vi "氨氮通讯.vi"() -> ()   [LabVIEW 2016, in "氨氮.lvlib"]
uses:
  <vilib>/Utility/config.llb/Write Key (Boolean).vi
  <vilib>/Utility/config.llb/Write Key (String).vi
  <vilib>/Utility/config.llb/Read Key (Boolean).vi
  <vilib>/Utility/config.llb/Read Key (String).vi
  <vilib>/Plasmionique/MB Master/MB_Master/MB_Master.lvclass
  <vilib>/Utility/config.llb/NI_LVConfig.lvlib
  <vilib>/Plasmionique/MB Master/MB Master.lvlib
  <vilib>/ptbypt/NI_PtbyPt.lvlib
panel:
  out "序列号":string
  out "状态告警区":T1
  out "测量数据区":T2 {"单位" items=["ug/L", "mg/L", "ppm", "mg/m3", "cm", "ppb", "ug/m3", "%", "nmol/mol", "umol/mol", "MPN/L", "MPN/100ml", "ng/m3", "NTU", "无量纲", "ms/cm", "us/cm", "℃", "mV", "万个/L"]}
  out "status":bool
  out "关键参数区":T3
  in  "读关键参数区":bool
  in  "读状态告警区":bool
  in  "读测量数据区":bool
  in  "站号":u16(ring) items=["总磷"=1, "氨氮"=3]
  in  "停止":bool
  in  "启动":bool
  in  "控制命令":u16(ring) items=["启动测量"=1, "标样核查"=2, "零点核查"=3, "跨度核查"=4, "空白测试"=5, "平行样测试"=6, "加标回收"=7, "空白校准"=8, "标样校准"=9, "初始化（清洗）"=10, "停止测试"=11, "仪器重启"=12, "校时"=13, "模式设置"=14, "测量间隔设置"=15]
  in  "控制命令参数":u16[](array[numeric]) format="%04xH"
  in  "VISA Resource":refnum<visa-resource-name>
  in  "启用模块":bool
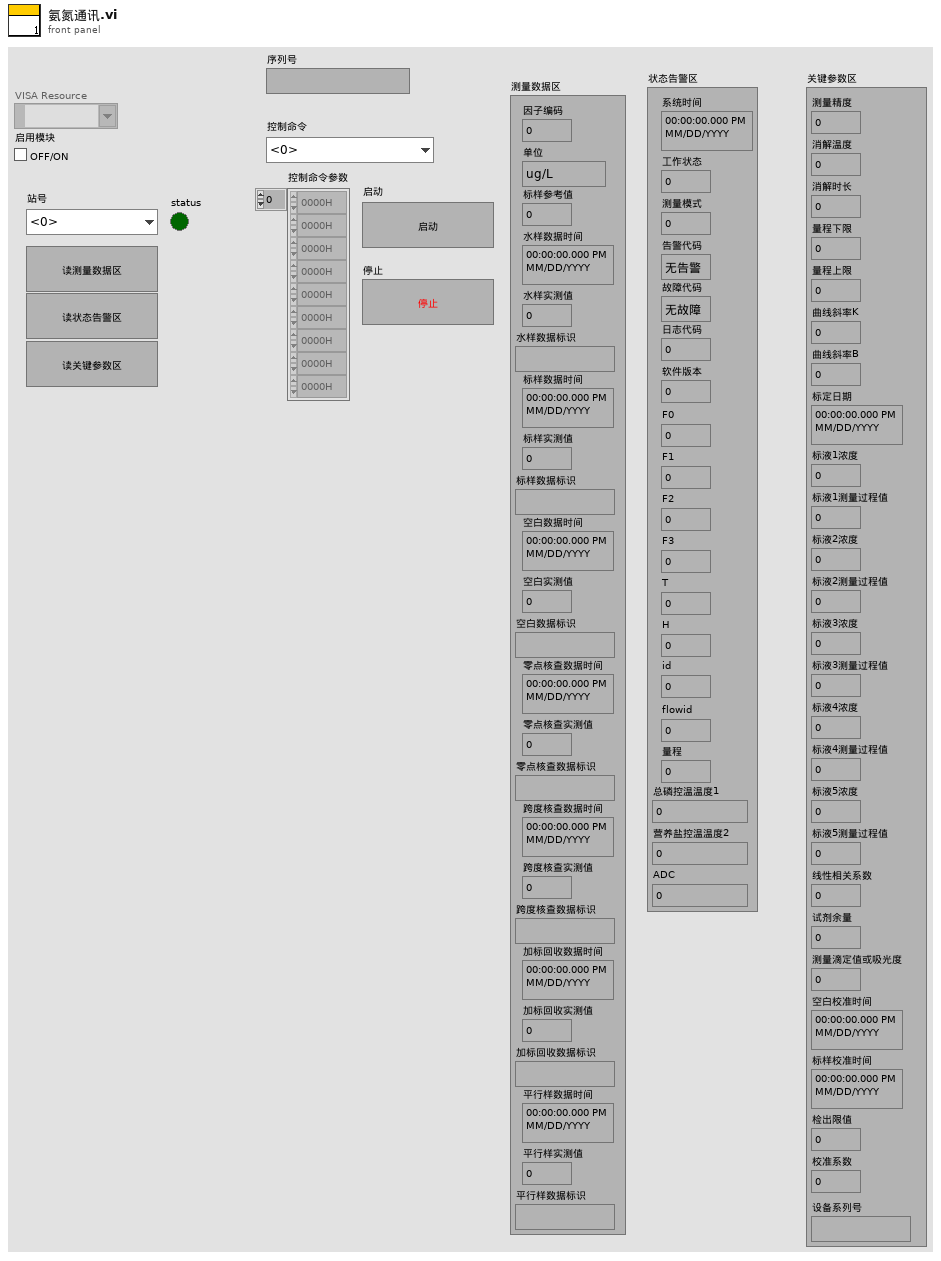
[diagram p1: front panel]
types:
  T1 = cluster{"系统时间":timestamp, "工作状态":u16, "测量模式":u16, "告警代码":enum16{"无告警", "缺试剂告警", "缺水样告警", "缺蒸馏水告警", "缺标液告警", "仪表漏液告警", "标定异常告警", "超量程告警", "加热异常", "低试剂预警", "超上限告警", "超下限告警", "仪表内部其他异常", "滴定异常告警", "电极异常告警", "量程切换告警", "参数设置告警", "PH电极电位异常", "电导率电极异常", "浊度光度异常", "溶解氧电极异常", "溶解氧光强异常", "温度异常告警", "PH异常告警", "溶解氧异常告警", "电导率异常告警", "浊度异常告警", "叶绿素异常告警", "藻密度异常告警", "蓝绿藻异常告警", "ORP异常告警", "氨氮异常告警", "清洁刷异常告警", "SD卡异常告警", "蓝牙异常告警", "Wifi异常告警", "流程异常告警"}, "故障代码":enum16{"无故障", "电机故障", "温度故障", "通讯故障", "滴定故障"}, "日志代码":u16, "软件版本":u16, "F0":sgl, "F1":sgl, "F2":sgl, "F3":sgl, "T":sgl, "H":sgl, "id":u16, "flowid":u16, "量程":u16, "ADC":sgl, "营养盐控温温度2":sgl, "总磷控温温度1":sgl}
  T2 = cluster{"因子编码":u32, "单位":u16, "标样参考值":sgl, "水样数据时间":timestamp, "水样实测值":sgl, "水样数据标识":string, "标样数据时间":timestamp, "标样实测值":sgl, "标样数据标识":string, "空白数据时间":timestamp, "空白实测值":sgl, "空白数据标识":string, "零点核查数据时间":timestamp, "零点核查实测值":sgl, "零点核查数据标识":string, "跨度核查数据时间":timestamp, "跨度核查实测值":sgl, "跨度核查数据标识":string, "加标回收数据时间":timestamp, "加标回收实测值":sgl, "加标回收数据标识":string, "平行样数据时间":timestamp, "平行样实测值":sgl, "平行样数据标识":string}
  T3 = cluster{"测量精度":u16, "消解温度":u16, "消解时长":u16, "量程下限":sgl, "量程上限":sgl, "曲线斜率K":sgl, "曲线斜率B":sgl, "标定日期":timestamp, "标液1浓度":sgl, "标液1测量过程值":sgl, "标液2浓度":sgl, "标液2测量过程值":sgl, "标液3浓度":sgl, "标液3测量过程值":sgl, "标液4浓度":sgl, "标液4测量过程值":sgl, "标液5浓度":sgl, "标液5测量过程值":sgl, "线性相关系数":sgl, "试剂余量":u32, "测量滴定值或吸光度":sgl, "空白校准时间":timestamp, "标样校准时间":timestamp, "检出限值":sgl, "校准系数":sgl, "设备系列号":string}
  T4 = typedef "NI_LVConfig.lvlib/Config Data RefNum.ctl" = refnum<k1>
  T5 = enum8{"Enabled", "Disabled", "Disabled and Grayed Out"}
  T6 = cluster{"系统时间":timestamp, "工作状态":enum16{"空闲", "水样测试", "标样核查", "零点核查", "跨度核查", "空白测试", "平行样测试", "加标回收", "空白校准", "标样校准", "初始化（清洗）"}, "测量模式":enum16{"待机", "连续模式", "周期模式", "定点模式", "受控模式", "手动模式"}, "告警代码":enum16{"无告警", "缺试剂告警", "缺水样告警", "缺蒸馏水告警", "缺标液告警", "仪表漏液告警", "标定异常告警", "超量程告警", "加热异常", "低试剂预警", "超上限告警", "超下限告警", "仪表内部其他异常", "滴定异常告警", "电极异常告警", "量程切换告警", "参数设置告警", "PH电极电位异常", "电导率电极异常", "浊度光度异常", "溶解氧电极异常", "溶解氧光强异常", "温度异常告警", "PH异常告警", "溶解氧异常告警", "电导率异常告警", "浊度异常告警", "叶绿素异常告警", "藻密度异常告警", "蓝绿藻异常告警", "ORP异常告警", "氨氮异常告警", "清洁刷异常告警", "SD卡异常告警", "蓝牙异常告警", "Wifi异常告警", "流程异常告警"}, "故障代码":enum16{"无故障", "电机故障", "温度故障", "通讯故障", "滴定故障"}, "日志代码":u16, "软件版本":u16, "F0":sgl, "F1":sgl, "F2":sgl, "F3":sgl, "T":sgl, "H":sgl, "id":u16, "flowid":u16, "量程":u16, "总磷控温温度1":sgl, "营养盐控温温度2":sgl, "ADC":sgl}
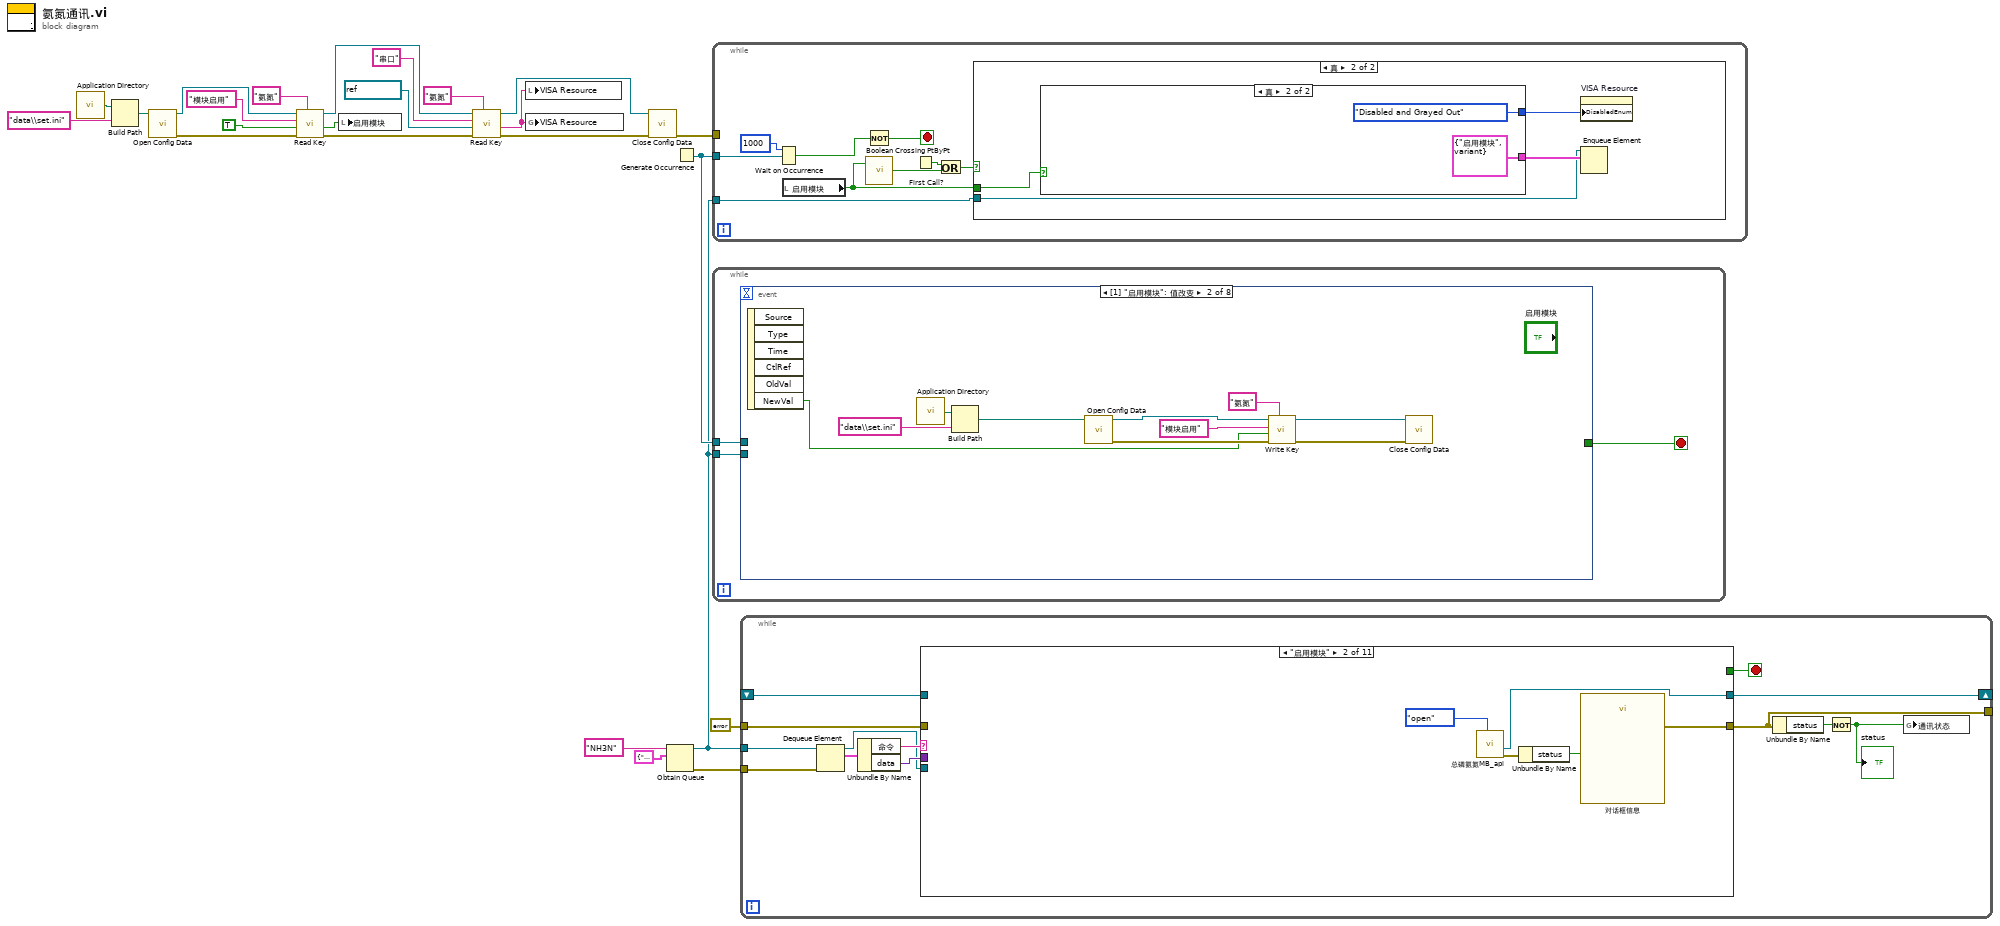
[diagram p0: block diagram]
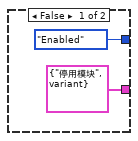
[diagram p3: hidden frame]
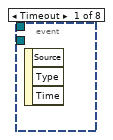
[diagram p4: hidden frame]
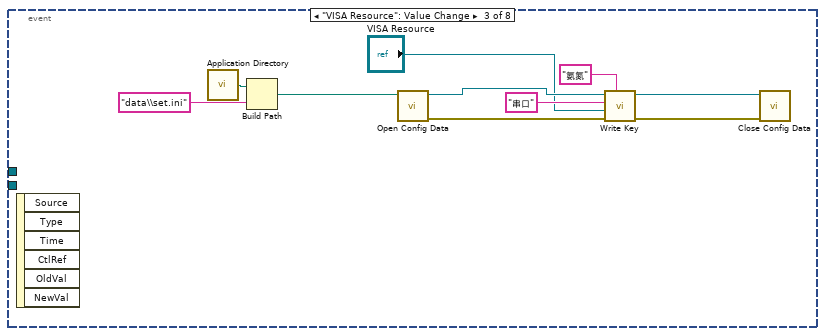
[diagram p5: hidden frame]
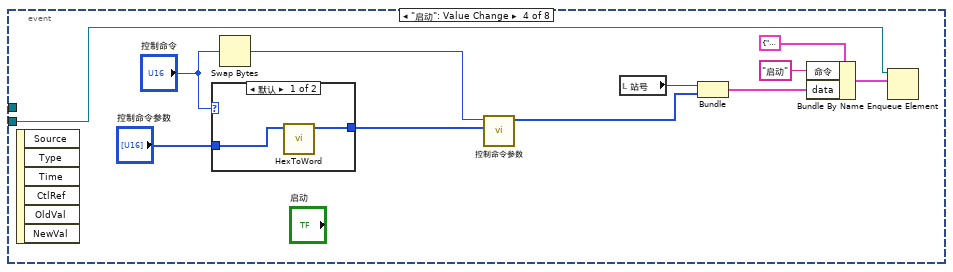
[diagram p6: hidden frame]
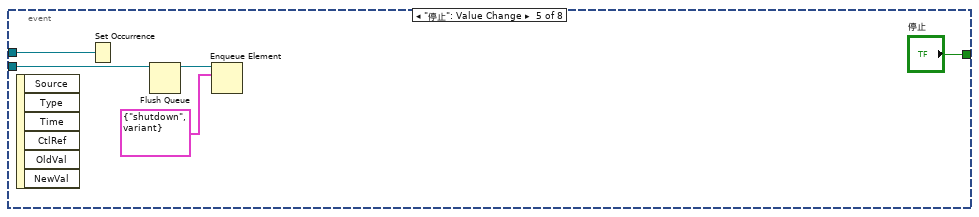
[diagram p8: hidden frame]
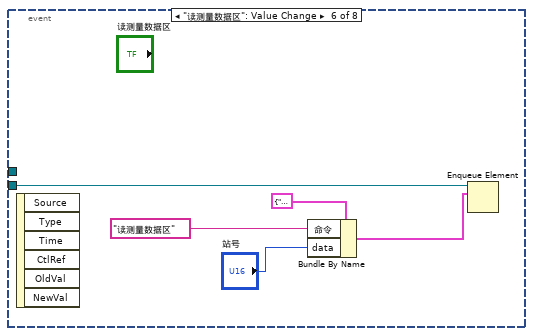
[diagram p9: hidden frame]
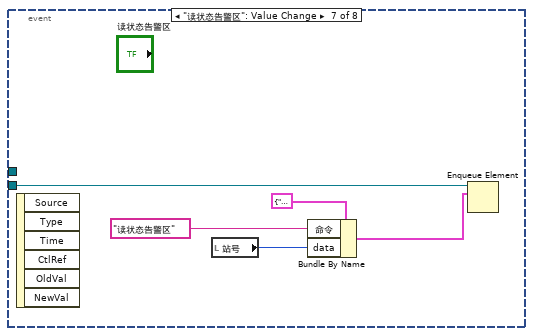
[diagram p10: hidden frame]
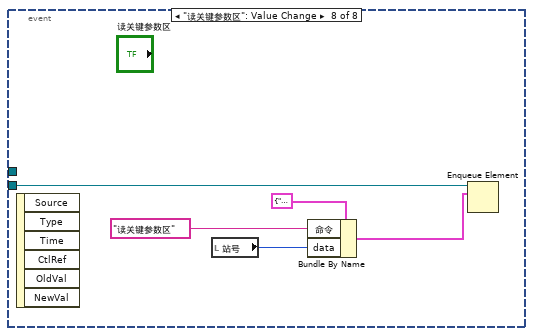
[diagram p11: hidden frame]
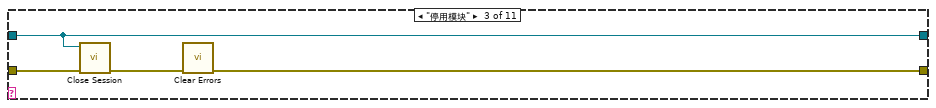
[diagram p13: hidden frame]
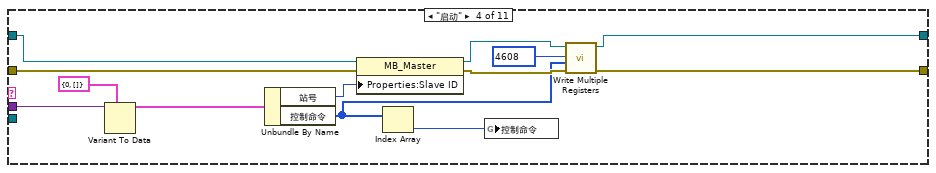
[diagram p14: hidden frame]
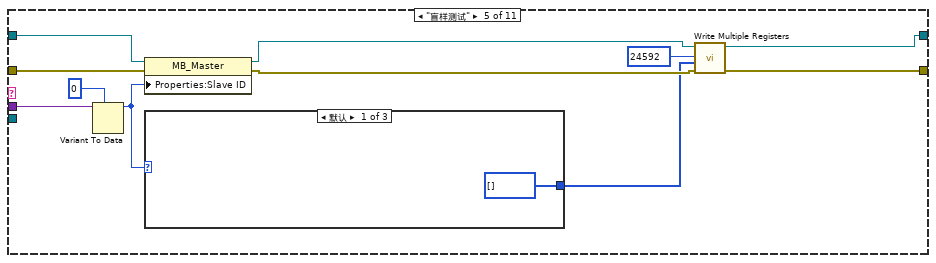
[diagram p15: hidden frame]
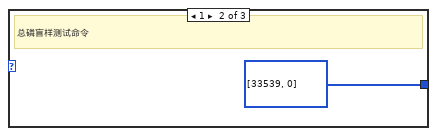
[diagram p16: hidden frame]
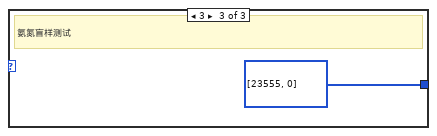
[diagram p17: hidden frame]
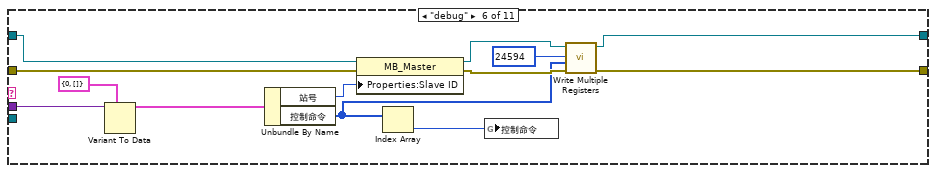
[diagram p18: hidden frame]
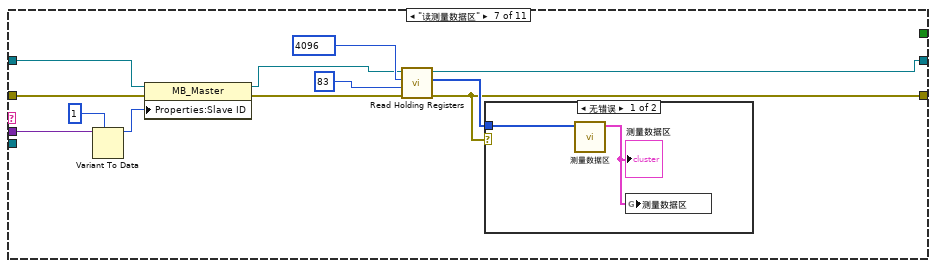
[diagram p19: hidden frame]
diagram:
  n1 = call <vilib>:"Application Directory.vi"() -> ("Application Directory"=w12:path)
  n2 = Build Path(base path=w12, name or relative path="data\\set.ini" ("名称或相对路径")) -> (appended path=w13:path)
  n3 = call <vilib>:"Open Config Data.vi"("configuration file path"=w13) -> ("error out"=w18:errorcluster, "refnum"=w17:T4)  [unwired: 8 in, 1 out]
  n4 = call-poly <vilib>:"Read Key.vi"("section"="氨氮", "error in (no error)"=w18, "default value"=TRUE ("启用模块"), "key"="模块启用", "refnum"=w17) -> ("error out"=w7:errorcluster, "value"=w10:bool, "refnum out"=w9:T4)  [unwired: 3 in, 1 out]
  n5 = local write "启用模块"(w10) -> ()
  n6 = call-poly <vilib>:"Read Key.vi"("section"="氨氮", "error in (no error)"=w7, "default value"=refnum<visa-resource-name> "COM7" ("VISA Resource"), "key"="串口", "refnum"=w9) -> ("error out"=w6:errorcluster, "value"=w2:string, "refnum out"=w8:T4)  [unwired: 3 in, 1 out]
  n7 = local write "VISA Resource"(w2) -> ()
  n8 = global write "VAR氨氮全局变量.vi" "VISA Resource"(w2) -> ()
  n9 = call <vilib>:"Close Config Data.vi"("error in (no error)"=w6, "refnum"=w8) -> ("error out"=w1:errorcluster)  [unwired: 8 in, 1 out]
  n10 = Obtain Queue(name (unnamed)="NH3N" ("名称（未命名）"), element data type=cluster{"命令":string, "data":variant} {"命令"="", "data"=variant}) -> (queue out=w19:refnum<queue>, error out=w22:errorcluster)  [unwired: 3 in, 1 out]
  n11 = Generate Occurrence() -> (w20:refnum<k4>)
  n12 = while {
    tunnel: w20 -> [w33]
    tunnel: w19 -> [w28]
    tunnel: w1 -> [_]
    stop <- w30 stop-if-true
    n13 = Wait on Occurrence(2:w33, 3:1000 ("毫秒超时(-1)")) -> (0:w31:bool)  [unwired: 1 in]
    n14 = local read "启用模块"() -> (w29:bool)
    n15 = Not(x=w31) -> (.not. x?=w30:bool)
    n16 = call <vilib>:"Boolean Crossing PtByPt.vi"("input"=w29) -> ("crossing"=w26:bool)  [unwired: 2 in]
    n17 = First Call?() -> (First Call?: T/F=w27:bool)
    n18 = Or(x=w27, y=w26) -> (x .or. y?=w25:bool)
    n19 = case shown="真" w25 {
      tunnel: w29 -> [_ w36]
      tunnel: w28 -> [_ w35]
      frame False {
      }
      frame True {
        n20 = case shown="真" w36 {
          tunnel: [cluster{"命令":string, "data":variant} {"命令"="停用模块", "data"=variant} ("元素") cluster{"命令":string, "data":variant} {"命令"="启用模块", "data"=variant} ("元素")] -> w37
          tunnel: [T5."Enabled" ("禁用") T5."Disabled and Grayed Out" ("禁用")] -> w34
          frame False {
          }
          frame True {
          }
        }
        n21 = property on="VISA Resource" class="VISAName"("DisabledEnum"=w34) -> ()  [unwired: 2 in, 2 out]
        n22 = Enqueue Element(queue=w35, element=w37) -> ()  [unwired: 2 in, 3 out]
      }
    }
  }
  n23 = while {
    tunnel: w19 -> [w44]
    tunnel: w20 -> [w42]
    stop <- w43 stop-if-true
    n24 = event shown="[1] \"启用模块\": 值改变" {
      selector: _ -> [_ _ _ _ _ _ _ _]
      dyn-events: _ -> [_ _ _ _ _ _ _ _]
      timeout: _ -> [_ _ _ _ _ _ _ _]
      tunnel: w44 -> [_ _ _ w75 w82 w88 w93 w98]
      tunnel: [_ _ _ _ "停止" _ _ _] -> w43
      tunnel: w42 -> [_ _ _ _ w79 _ _ _]
      event Timeout {
        n25 = event-data() -> ()  [unwired: 1 in, 3 out]
      }
      event "启用模块": Value Change {
        n26 = event-data() -> ("NewVal"=w45:bool)  [unwired: 1 in, 5 out]
        n27 = call <vilib>:"Application Directory.vi"() -> ("Application Directory"=w47:path)
        n28 = Build Path(base path=w47, name or relative path="data\\set.ini" ("名称或相对路径")) -> (appended path=w48:path)
        n29 = call <vilib>:"Open Config Data.vi"("configuration file path"=w48) -> ("error out"=w54:errorcluster, "refnum"=w53:T4)  [unwired: 8 in, 1 out]
        n30 = call-poly <vilib>:"Write Key.vi"("section"="氨氮", "error in (no error)"=w54, "value"=w45, "key"="模块启用", "refnum"=w53) -> ("error out"=w50:errorcluster, "refnum out"=w46:T4)  [unwired: 4 in, 1 out]
        n31 = call <vilib>:"Close Config Data.vi"("error in (no error)"=w50, "refnum"=w46) -> ()  [unwired: 8 in, 2 out]
      }
      event "VISA Resource": Value Change {
        n32 = event-data() -> ()  [unwired: 1 in, 6 out]
        n33 = call <vilib>:"Application Directory.vi"() -> ("Application Directory"=w57:path)
        n34 = Build Path(base path=w57, name or relative path="data\\set.ini" ("名称或相对路径")) -> (appended path=w58:path)
        n35 = call <vilib>:"Open Config Data.vi"("configuration file path"=w58) -> ("error out"=w64:errorcluster, "refnum"=w63:T4)  [unwired: 8 in, 1 out]
        n36 = call-poly <vilib>:"Write Key.vi"("section"="氨氮", "error in (no error)"=w64, "value"="VISA Resource", "key"="串口", "refnum"=w63) -> ("error out"=w60:errorcluster, "refnum out"=w56:T4)  [unwired: 4 in, 1 out]
        n37 = call <vilib>:"Close Config Data.vi"("error in (no error)"=w60, "refnum"=w56) -> ()  [unwired: 8 in, 2 out]
      }
      event "启动": Value Change {
        n38 = event-data() -> ()  [unwired: 1 in, 6 out]
        n39 = case shown="默认" "控制命令" {
          tunnel: "控制命令参数" -> [w77 w78]
          tunnel: [w76 w78] -> w65
          frame Default {
            n40 = call "HexToWord.vi"("数组"=w77) -> ("WORD"=w76:u16[])  [unwired: 10 in]
          }
          frame 13 {
          }
        }
        n41 = Swap Bytes(anything="控制命令") -> (byte swapped=w68:u16)
        n42 = call "控制命令参数.vi"("控制命令参数"=w65, "控制命令"=w68) -> ("控制命令输出"=w71:u16[])  [unwired: 9 in]
        n43 = local read "站号"() -> (w70:u16)
        n44 = Bundle("站号"=w70, "控制命令输出"=w71) -> (w69:cluster{"站号":u16, "控制命令输出":u16[]})  [unwired: 1 in]
        n45 = Bundle By Name(cluster=cluster{"命令":string, "data":variant} {"命令"="", "data"=variant} ("元素"), "命令"="启动", "data"=w69) -> (w73:cluster{"命令":string, "data":variant})
        n46 = Enqueue Element(queue=w75, element=w73) -> ()  [unwired: 2 in, 3 out]
      }
      event "停止": Value Change {
        n47 = event-data() -> ()  [unwired: 1 in, 6 out]
        n48 = Set Occurrence(w79) -> ()
        n49 = Flush Queue(queue=w82) -> (queue out=w81:refnum<queue>)  [unwired: 1 in, 2 out]
        n50 = Enqueue Element(queue=w81, element=cluster{"命令":string, "data":variant} {"命令"="shutdown", "data"=variant} ("元素")) -> ()  [unwired: 2 in, 3 out]
      }
      event "读测量数据区": Value Change {
        n51 = event-data() -> ()  [unwired: 1 in, 6 out]
        n52 = Bundle By Name(cluster=cluster{"命令":string, "data":variant} {"命令"="", "data"=variant} ("元素"), "命令"="读测量数据区", "data"="站号") -> (w86:cluster{"命令":string, "data":variant})
        n53 = Enqueue Element(queue=w88, element=w86) -> ()  [unwired: 2 in, 3 out]
      }
      event "读状态告警区": Value Change {
        n54 = event-data() -> ()  [unwired: 1 in, 6 out]
        n55 = local read "站号"() -> (w89:u16)
        n56 = Bundle By Name(cluster=cluster{"命令":string, "data":variant} {"命令"="", "data"=variant} ("元素"), "命令"="读状态告警区", "data"=w89) -> (w91:cluster{"命令":string, "data":variant})
        n57 = Enqueue Element(queue=w93, element=w91) -> ()  [unwired: 2 in, 3 out]
      }
      event "读关键参数区": Value Change {
        n58 = event-data() -> ()  [unwired: 1 in, 6 out]
        n59 = local read "站号"() -> (w94:u16)
        n60 = Bundle By Name(cluster=cluster{"命令":string, "data":variant} {"命令"="", "data"=variant} ("元素"), "命令"="读关键参数区", "data"=w94) -> (w96:cluster{"命令":string, "data":variant})
        n61 = Enqueue Element(queue=w98, element=w96) -> ()  [unwired: 2 in, 3 out]
      }
    }
  }
  n62 = while {
    tunnel: w19 -> [w111]
    tunnel: w22 -> [w110]
    shift-right: [w108] -> _
    shift-left: _ -> [w107]
    tunnel: errorcluster {"status"=FALSE, "code"=0, "source"=""} ("error out") -> [w106]
    tunnel: [w101] -> _
    stop <- w109 stop-if-true
    n63 = Dequeue Element(queue=w111, error in (no error)=w110) -> (queue out=w102:refnum<queue>, element=w104:cluster{"命令":string, "data":variant})  [unwired: 1 in, 2 out]
    n64 = Unbundle By Name(w104) -> ("命令"=w105:string, "data"=w103:variant)
    n65 = case shown="\"启用模块\"" w105 {
      tunnel: w103 -> [_ _ _ w132 w143 w160 w169 w179 w194 w208 _]
      tunnel: w102 -> [_ _ _ _ _ _ _ _ _ _ w221]
      tunnel: [_ _ _ _ _ _ _ _ _ _ TRUE] -> w109
      tunnel: [w112 w115 w119 w135 w146 w162 w174 w188 w201 w215 w217] -> w108
      tunnel: [w113 w117 w120 w134 w145 w161 w163 w189 w202 w216 w218] -> w101
      tunnel: w107 -> [w112 _ w119 w131 w142 w159 w168 w182 w197 w211 w217]
      tunnel: w106 -> [w113 _ w122 w128 w139 w156 w166 w183 w198 w212 w219]
      frame Default {
      }
      frame "启用模块" {
        n66 = call "总磷氨氮MB_api.vi"("STEP"=enum16{"open", "read", "write", "close"}."open") -> ("error out"=w114:errorcluster, "MB session out"=w115:refnum<class "MB_Master.lvclass">)  [unwired: 7 in, 2 out]
        n67 = Unbundle By Name(w114) -> ("status"=w118:bool)
        n68 = call "对话框信息"("Enable"=w118) -> ("error out"=w117:errorcluster)  [unwired: 9 in, 1 out]
      }
      frame "停用模块" {
        n69 = call-dynamic "Close Session.vi"("error in (no error)"=w122, "MB session in"=w119) -> ("error out"=w121:errorcluster)  [unwired: 9 in]
        n70 = call <vilib>:"Clear Errors.vi"("error in (no error)"=w121) -> ("error out"=w120:errorcluster)  [unwired: 5 in, 1 out]
      }
      frame "启动" {
        n71 = Variant To Data(type=cluster{"站号":u16, "控制命令":u16[]} {"站号"=0, "控制命令"=[]} ("输出簇"), Variant=w132) -> (data=w126:cluster{"站号":u16, "控制命令":u16[]})  [unwired: 1 in, 1 out]
        n72 = Unbundle By Name(w126) -> ("站号"=w125:u16, "控制命令"=w123:u16[])
        n73 = property class="MB_Master"(reference=w131, error in=w128, "Properties:Slave ID"=w125) -> (reference out=w130:refnum<class "MB_Master.lvclass">, error out=w129:errorcluster)
        n74 = Index Array(array=w123) -> (element=w124:u16)  [unwired: 1 in]
        n75 = global write "VAR氨氮全局变量.vi" "控制命令"(w124) -> ()
        n76 = call <vilib>:"Write Multiple Registers.vi"("error in (no error)"=w129, "values"=w123, "starting address"=u16 4608, "MB session in"=w130) -> ("error out"=w134:errorcluster, "MB session out"=w135:refnum<class "MB_Master.lvclass">)  [unwired: 6 in]
      }
      frame "盲样测试" {
        n77 = Variant To Data(type=0, Variant=w143) -> (data=w136:i32)  [unwired: 1 in, 1 out]
        n78 = property class="MB_Master"(reference=w142, error in=w139, "Properties:Slave ID"=w136) -> (reference out=w141:refnum<class "MB_Master.lvclass">, error out=w140:errorcluster)
        n79 = case shown="默认" w136 {
          tunnel: [u16[] [] ("values") u16[] [33539, 0] ("values") u16[] [23555, 0] ("values")] -> w138
          frame Default {
          }
          frame 1 {
            # "总磷盲样测试命令"
          }
          frame 3 {
            # "氨氮盲样测试"
          }
        }
        n80 = call <vilib>:"Write Multiple Registers.vi"("error in (no error)"=w140, "values"=w138, "starting address"=u16 24592, "MB session in"=w141) -> ("error out"=w145:errorcluster, "MB session out"=w146:refnum<class "MB_Master.lvclass">)  [unwired: 6 in]
      }
      frame "debug" {
        n81 = Variant To Data(type=cluster{"站号":u16, "控制命令":u16[]} {"站号"=0, "控制命令"=[]} ("输出簇"), Variant=w160) -> (data=w154:cluster{"站号":u16, "控制命令":u16[]})  [unwired: 1 in, 1 out]
        n82 = Unbundle By Name(w154) -> ("站号"=w153:u16, "控制命令"=w151:u16[])
        n83 = property class="MB_Master"(reference=w159, error in=w156, "Properties:Slave ID"=w153) -> (reference out=w158:refnum<class "MB_Master.lvclass">, error out=w157:errorcluster)
        n84 = Index Array(array=w151) -> (element=w152:u16)  [unwired: 1 in]
        n85 = global write "VAR氨氮全局变量.vi" "控制命令"(w152) -> ()
        n86 = call <vilib>:"Write Multiple Registers.vi"("error in (no error)"=w157, "values"=w151, "starting address"=u16 24594, "MB session in"=w158) -> ("error out"=w161:errorcluster, "MB session out"=w162:refnum<class "MB_Master.lvclass">)  [unwired: 6 in]
      }
      frame "读测量数据区" {
        n87 = Variant To Data(type=u8 1 ("Slave ID"), Variant=w169) -> (data=w170:u8)  [unwired: 1 in, 1 out]
        n88 = property class="MB_Master"(reference=w168, error in=w166, "Properties:Slave ID"=w170) -> (reference out=w167:refnum<class "MB_Master.lvclass">, error out=w165:errorcluster)
        n89 = call <vilib>:"Read Holding Registers.vi"("error in (no error)"=w165, "quantity"=u16 83, "starting address"=u16 4096, "MB session in"=w167) -> ("error out"=w163:errorcluster, "Registers"=w164:u16[], "MB session out"=w174:refnum<class "MB_Master.lvclass">)  [unwired: 5 in]
        n90 = case shown="无错误" w163 {
          tunnel: w164 -> [w176 _]
          frame No Error {
            n91 = call "测量数据区.vi"("数组"=w176) -> ("测量数据区"=w175:T2)  [unwired: 10 in]
            "测量数据区" <- w175
            n92 = global write "VAR氨氮全局变量.vi" "测量数据区"(w175) -> ()
          }
          frame Error {
          }
        }
      }
      frame "读状态告警区" {
        n93 = Variant To Data(type=u8 1 ("Slave ID"), Variant=w179) -> (data=w184:u8)  [unwired: 1 in, 1 out]
        n94 = property class="MB_Master"(reference=w182, error in=w183, "Properties:Slave ID"=w184) -> (reference out=w181:refnum<class "MB_Master.lvclass">, error out=w180:errorcluster)
        n95 = call <vilib>:"Read Holding Registers.vi"("error in (no error)"=w180, "quantity"=u16 24, "starting address"=u16 4224, "MB session in"=w181) -> ("error out"=w189:errorcluster, "Registers"=w178:u16[], "MB session out"=w188:refnum<class "MB_Master.lvclass">)  [unwired: 5 in]
        n96 = call "状态告警区.vi"("数组"=w178) -> ("状态告警区"=w177:T6)  [unwired: 10 in]
        "状态告警区" <- w177
        n97 = global write "VAR氨氮全局变量.vi" "状态告警区"(w177) -> ()
      }
      frame "读关键参数区" {
        n98 = Variant To Data(type=u8 1 ("Slave ID"), Variant=w194) -> (data=w192:u8)  [unwired: 1 in, 1 out]
        n99 = property class="MB_Master"(reference=w197, error in=w198, "Properties:Slave ID"=w192) -> (reference out=w196:refnum<class "MB_Master.lvclass">, error out=w195:errorcluster)
        n100 = call <vilib>:"Read Holding Registers.vi"("error in (no error)"=w195, "quantity"=u16 19, "starting address"=u16 4256, "MB session in"=w196) -> ("error out"=w202:errorcluster, "Registers"=w191:u16[], "MB session out"=w201:refnum<class "MB_Master.lvclass">)  [unwired: 5 in]
        n101 = call "关键参数区.vi"("数组"=w191) -> ("关键参数区"=w190:T3)  [unwired: 10 in]
        "关键参数区" <- w190
        n102 = global write "VAR氨氮全局变量.vi" "关键参数区"(w190) -> ()
      }
      frame "读序列号" {
        n103 = Variant To Data(type=u8 1 ("Slave ID"), Variant=w208) -> (data=w206:u8)  [unwired: 1 in, 1 out]
        n104 = property class="MB_Master"(reference=w211, error in=w212, "Properties:Slave ID"=w206) -> (reference out=w210:refnum<class "MB_Master.lvclass">, error out=w209:errorcluster)
        n105 = call <vilib>:"Read Holding Registers.vi"("error in (no error)"=w209, "quantity"=u16 6, "starting address"=u16 3, "MB session in"=w210) -> ("error out"=w216:errorcluster, "Registers"=w205:u16[], "MB session out"=w215:refnum<class "MB_Master.lvclass">)  [unwired: 5 in]
        n106 = call "HexToString.vi"("数组"=w205) -> ("STRING"=w204:string[])  [unwired: 10 in]
        n107 = Index Array(array=w204) -> (element=w203:string)  [unwired: 1 in]
        "序列号" <- w203
        n108 = global write "VAR氨氮全局变量.vi" "序列号"(w203) -> ()
      }
      frame "shutdown" {
        n109 = call-dynamic "Close Session.vi"("error in (no error)"=w219, "MB session in"=w217) -> ("error out"=w218:errorcluster)  [unwired: 9 in]
        n110 = Flush Queue(queue=w221) -> (queue out=w220:refnum<queue>)  [unwired: 1 in, 2 out]
        n111 = Release Queue(queue=w220) -> ()  [unwired: 2 in, 3 out]
      }
    }
    n112 = Unbundle By Name(w101) -> ("status"=w100:bool)
    n113 = Not(x=w100) -> (.not. x?=w99:bool)
    "status" <- w99
    n114 = global write "VAR氨氮全局变量.vi" "通讯状态"(w99) -> ()
  }
